vi "Untitled 1.vi"() -> ()   [LabVIEW 2011]
uses:
  JSON Value/JSON Value.lvclass
  JSON Array/JSON Array.lvclass
panel:
  out "offset":i32
  out "String 2":string
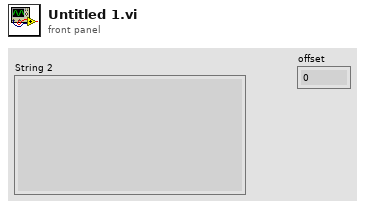
[diagram p1: front panel]
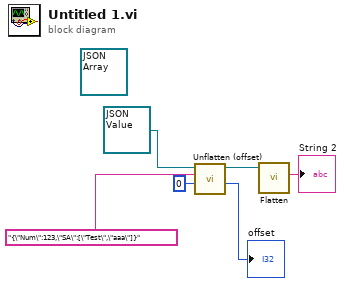
[diagram p0: block diagram]
diagram:
  (unwired) refnum<class "JSON Array.lvclass"> refnum ("JSON Array.lvclass")
  n1 = call-dynamic "Unflatten (offset).vi"("offset (0)"=0, "JSON stream"="{\"Num\":123,\"SA\":[\"Test\",\"aaa\"]}" ("String"), "JSON Value in"=refnum<class "JSON Value.lvclass"> refnum) -> ("offset"=→"offset":i32, "JSON Value out"=w4:refnum<class "JSON Value.lvclass">)  [unwired: 5 in, 2 out]
  n2 = call-dynamic "Flatten.vi"("JSON Value in"=w4) -> ("String"=→"String 2":string)  [unwired: 9 in, 1 out]
